vi "Data Stream Control (Additive).vi"(4 "ready for input?":bool=TRUE, 5 "stream.additive num samples 0":u16, 7 "stream.request state 0":T1, 9 "data valid":bool=TRUE caption="data valid (true)", 10 "element count":u16=1 caption="element count (1)") -> (0 "permissed elements":u16, 1 "send data":bool, 2 "stream.state 0":T1, 3 "stream.samples transferred 0":u64, 6 "force data":bool)   [LabVIEW 2015, in "niInstr Streaming v1 FPGA.lvlib"]
doc: "Similar to Data Stream Control, this VI is intended for use in additive stream functions. It is primarily an implementation detail of helping to split the stream control between \"fast\" data interface loops and \"slow\" data control/processing loops.\n\nSee examples for details of usage."
uses:
  <instrlib>/_niInstr/Streaming/v1/FPGA/niInstr Streaming v1 FPGA.lvlib
  <instrlib>/_niInstr/Streaming/v1/Common/Stream State.ctl
  <instrlib>/_niInstr/Streaming/v1/Common/niInstr Streaming v1 Common.lvlib
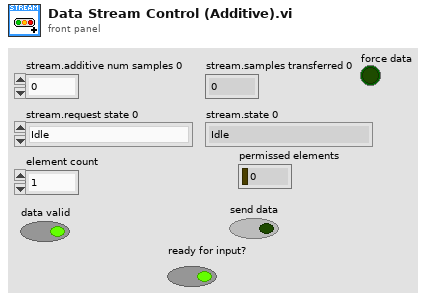
[diagram p1: front panel]
types:
  T1 = typedef "niInstr Streaming v1 Common.lvlib/Stream State.ctl" = enum8{"Idle", "Finite Transfer", "Continuous", "Done", "Error", "Not Ready", "Cancel"}
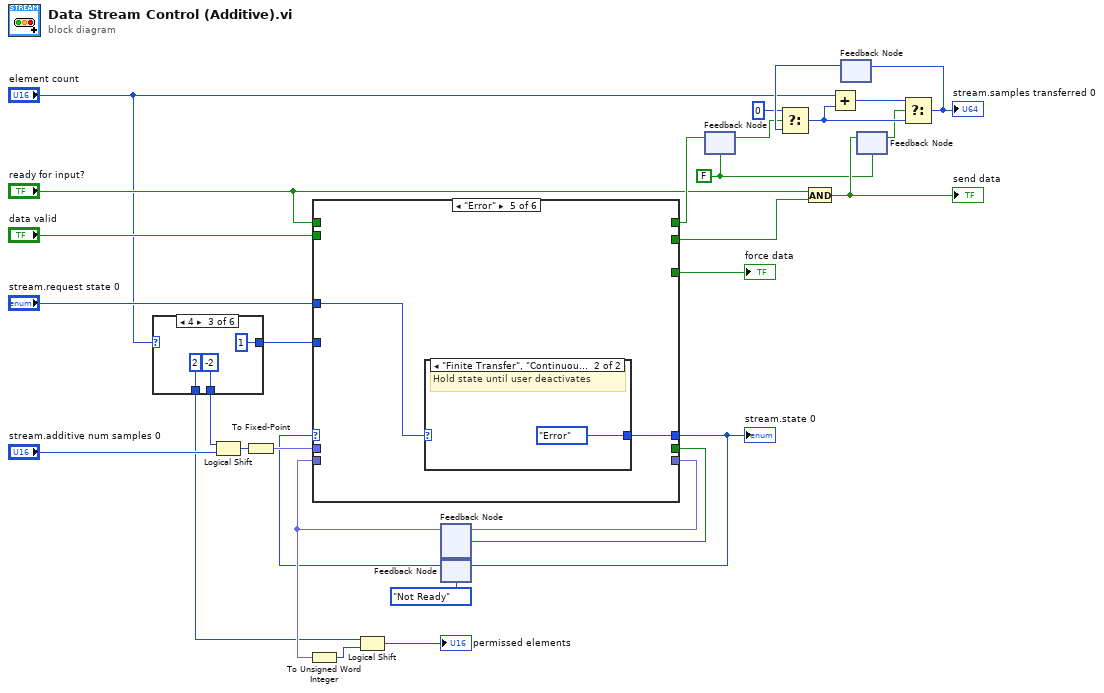
[diagram p0: block diagram]
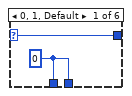
[diagram p2: hidden frame]
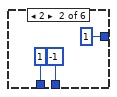
[diagram p3: hidden frame]
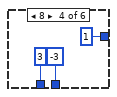
[diagram p4: hidden frame]
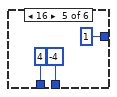
[diagram p5: hidden frame]
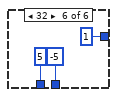
[diagram p6: hidden frame]
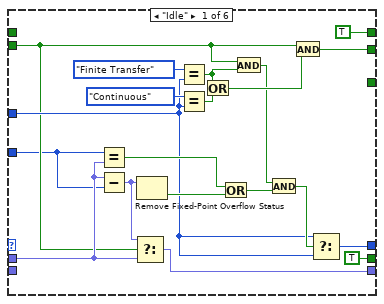
[diagram p7: hidden frame]
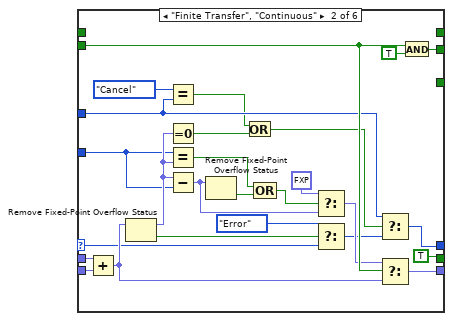
[diagram p8: hidden frame]
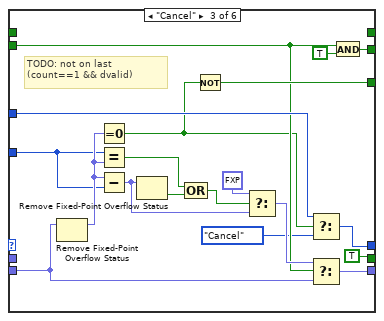
[diagram p9: hidden frame]
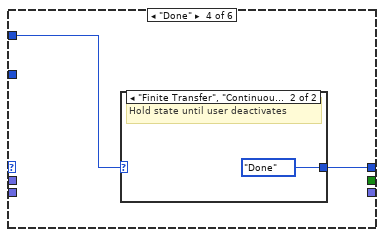
[diagram p10: hidden frame]
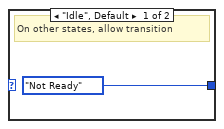
[diagram p12: hidden frame]
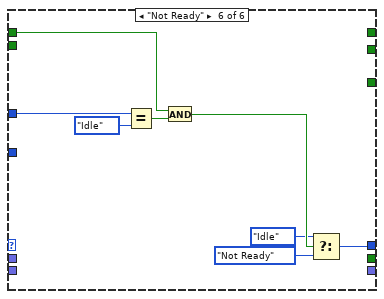
[diagram p13: hidden frame]
diagram:
  w3 = FALSE
  n1 = case shown="4" "element count" {
    selector: "element count" -> [w32 _ _ _ _ _]
    tunnel: [w32 u16 1 ("Element Count") u16 1 ("Element Count") u16 1 ("Element Count") u16 1 ("Element Count") u16 1 ("Element Count")] -> w11
    tunnel: [w31 i16 -1 ("y") i16 -2 ("y") i16 -3 ("y") i16 -4 ("y") i16 -5 ("y")] -> w8
    tunnel: [w31 i16 1 ("y") i16 2 ("y") i16 3 ("y") i16 4 ("y") i16 5 ("y")] -> w4
    frame 0, 1, Default {
      w31 = i16 0 ("y")
    }
    frame 2 {
    }
    frame 4 {
    }
    frame 8 {
    }
    frame 16 {
    }
    frame 32 {
    }
  }
  n2 = Logical Shift(y=w8, x="stream.additive num samples 0") -> (x << y=w10:u16)
  n3 = To Fixed-Point(number=w10) -> (fixed-point=w24:fxp<+,10,10>)  [unwired: 1 in]
  n4 = feedback #1() -> (w7:fxp<+,10,10>)  [unwired: 1 in]
  n5 = To Unsigned Word Integer(number=w7) -> (unsigned 16bit integer=w6:u16)
  n6 = Logical Shift(y=w4, x=w6) -> (x << y=→"permissed elements":u16)
  n7 = feedback #2(Stream_State."Not Ready" ("stream.state 0")) -> (w2:T1)
  n8 = case shown="\"Error\"" w2 {
    selector: w2 -> [_ w69 _ _ _ _]
    tunnel: [w64 w92 w111 w113 w117 w128] -> w1
    tunnel: "stream.request state 0" -> [w53 w75 w102 w114 w118 w127]
    tunnel: "data valid" -> [w51 w84 w100 _ _ _]
    tunnel: [w52 w89 w109 _ _ _] -> w28
    tunnel: [TRUE _ _ _ _ _] -> w25
    tunnel: w24 -> [w55 w88 _ _ _ _]
    tunnel: [w54 w78 w104 _ _ _] -> w23
    tunnel: w7 -> [_ w91 w96 _ _ _]
    tunnel: "ready for input?" -> [_ _ _ _ _ w124]
    tunnel: w11 -> [w48 w72 w94 _ _ _]
    tunnel: [TRUE TRUE TRUE _ _ _] -> w20
    tunnel: [_ _ w101 _ _ _] -> w19
    frame "Idle" {
      n9 = Equal?(x=w48, y=w55) -> (x = y?=w58:bool)
      n10 = Subtract(x=w55, y=w48) -> (x-y=w56:fxp<+,10,10>)
      n11 = Select(t=w56, s=w51, f=w55) -> (s? t:f=w54:fxp<+,10,10>)
      n12 = Remove Fixed-Point Overflow Status(3:w56) -> (0:w66:bool)  [unwired: 1 out]
      n13 = Equal?(x=Stream_State."Finite Transfer", y=w53) -> (x = y?=w50:bool)
      n14 = Equal?(x=Stream_State."Continuous", y=w53) -> (x = y?=w59:bool)
      n15 = Or(x=w50, y=w59) -> (x .or. y?=w60:bool)
      n16 = Or(x=w58, y=w66) -> (x .or. y?=w65:bool)
      n17 = And(x=w51, y=w50) -> (x .and. y?=w49:bool)
      n18 = And(x=w49, y=w65) -> (x .and. y?=w63:bool)
      n19 = And(x=w51, y=w60) -> (x .and. y?=w52:bool)
      n20 = Select(t=w53, s=w63, f=w53) -> (s? t:f=w64:T1)
    }
    frame "Finite Transfer", "Continuous" {
      n21 = Add(x=w88, y=w91) -> (x+y=w85:fxp<+,10,10>)
      n22 = Remove Fixed-Point Overflow Status(3:w85) -> (0:w70:bool, 1:w79:fxp<+,10,10>)
      n23 = Equal?(x=Stream_State."Cancel", y=w75) -> (x = y?=w73:bool)
      n24 = Equal To 0?(x=w79) -> (x = 0?=w81:bool)
      n25 = Equal?(x=w72, y=w79) -> (x = y?=w90:bool)
      n26 = Subtract(x=w79, y=w72) -> (x-y=w77:fxp<+,10,10>)
      n27 = Remove Fixed-Point Overflow Status(3:w77) -> (0:w93:bool)  [unwired: 1 out]
      n28 = Or(x=w73, y=w81) -> (x .or. y?=w76:bool)
      n29 = Compound Arithmetic op=OR(w90, w93) -> (w83:bool)
      n30 = Select(t=fxp<+,10,10> 0.0, s=w83, f=w77) -> (s? t:f=w80:fxp<+,10,10>)
      n31 = Select(t=Stream_State."Error", s=w70, f=w69) -> (s? t:f=w68:T1)
      n32 = Select(t=w75, s=w76, f=w68) -> (s? t:f=w92:T1)
      n33 = Select(t=w80, s=w84, f=w85) -> (s? t:f=w78:fxp<+,10,10>)
      n34 = And(x=w84, y=TRUE) -> (x .and. y?=w89:bool)
    }
    frame "Cancel" {
      # "TODO: not on last \n(count==1 && dvalid)"
      n35 = Remove Fixed-Point Overflow Status(3:w96) -> (1:w95:fxp<+,10,10>)  [unwired: 1 out]
      n36 = Equal To 0?(x=w95) -> (x = 0?=w97:bool)
      n37 = Equal?(x=w94, y=w95) -> (x = y?=w110:bool)
      n38 = Subtract(x=w95, y=w94) -> (x-y=w103:fxp<+,10,10>)
      n39 = Remove Fixed-Point Overflow Status(3:w103) -> (0:w112:bool)  [unwired: 1 out]
      n40 = Compound Arithmetic op=OR(w110, w112) -> (w98:bool)
      n41 = Not(x=w97) -> (.not. x?=w101:bool)
      n42 = Select(t=fxp<+,10,10> 0.0, s=w98, f=w103) -> (s? t:f=w105:fxp<+,10,10>)
      n43 = Select(t=w102, s=w97, f=Stream_State."Cancel" ("x")) -> (s? t:f=w111:T1)
      n44 = Select(t=w105, s=w100, f=w96) -> (s? t:f=w104:fxp<+,10,10>)
      n45 = And(x=w100, y=TRUE) -> (x .and. y?=w109:bool)
    }
    frame "Done" {
      n46 = case shown="\"Finite Transfer\", \"Continuous\"" w114 {
        selector: w114 -> [w115 _]
        tunnel: [w115 Stream_State."Done" ("stream.state 0")] -> w113
        frame "Idle", Default {
          # "On other states, allow transition"
        }
        frame "Finite Transfer", "Continuous" {
          # "Hold state until user deactivates"
        }
      }
    }
    frame "Error" {
      n47 = case shown="\"Finite Transfer\", \"Continuous\", \"Error\"" w118 {
        tunnel: [Stream_State."Not Ready" ("f") Stream_State."Error" ("stream.state 0")] -> w117
        frame "Idle", Default {
          # "On other states, allow transition"
        }
        frame "Finite Transfer", "Continuous", "Error" {
          # "Hold state until user deactivates"
        }
      }
    }
    frame "Not Ready" {
      n48 = Equal?(x=w127, y=Stream_State."Idle" ("stream.state 0")) -> (x = y?=w125:bool)
      n49 = And(x=w124, y=w125) -> (x .and. y?=w123:bool)
      n50 = Select(t=Stream_State."Idle" ("stream.state 0"), s=w123, f=Stream_State."Not Ready" ("stream.state 0")) -> (s? t:f=w128:T1)
    }
  }
  "stream.state 0" <- w1
  "force data" <- w19
  n51 = feedback-in #1(w23, w20) -> ()
  n52 = feedback-in #2(w1) -> ()
  n53 = feedback #3(w3) -> (w14:bool)
  n54 = feedback-in #3(w25) -> ()
  n55 = And(x="ready for input?", y=w28) -> (x .and. y?=w27:bool)
  "send data" <- w27
  n56 = feedback #4() -> (w16:u64)  [unwired: 1 in]
  n57 = Select(t=u64 0 ("f"), s=w14, f=w16) -> (s? t:f=w17:u64)
  n58 = Add(x="element count", y=w17) -> (x+y=w18:u64)
  n59 = feedback #5(w3) -> (w13:bool)
  n60 = feedback-in #5(w27) -> ()
  n61 = Select(t=w18, s=w13, f=w17) -> (s? t:f=w26:u64)
  "stream.samples transferred 0" <- w26
  n62 = feedback-in #4(w26) -> ()
